vi "VPI_Thresholds.vi"(0 "Circle Mask":bool, 2 "mask":sgl[][](array[numeric]), 4 "GThresholds":T1={"Vel Range"={1.4018691588785046, 50.0}, "PFlow Range"={22.429906542056074, 90.28037383177569}, "IQ Range"={28.037383177570092, 102.05607476635514}, "ShortLag"={33.08411214953271, 88.59813084112149}, "Mean Pow"={0.0, 41.12149532710281}, "powT"={0.0, 41.12149532710281}, "varT"={0.0, 41.12149532710281}} {"varT" scale=0.0..100.0; "powT" scale=0.0..100.0; "Mean Pow" scale=0.0..100.0; "ShortLag" scale=0.0..120.0; "IQ Range" scale=-25.0..120.0; "PFlow Range" scale=0.0..120.0; "Vel Range" scale=-1.0..150.0}, 6 "Datea items":T8={"Vector Refnum"=refnum, "Vector Image"=refnum, "Data Path"=path "", "abs(IQ)"=[], "Vector Complex"=[], "pow"=[], "Dimensions"={"xdim"=0.0, "ydim"=0.0, "zdim"=0.0, "skip"=0.0, "ensembleC"=0.0, "ensembleVar\n"=0.0, "#tx"=0.0, "#Rx"=0.0, "deltaX"=0.0, "deltaY"=0.0, "x start"=0.0, "ystart"=0.0}, "vars short lag"=[], "mean pow "=[], "mean var"=[], "Color Dop Refnum"=refnum, "Color Dop Image"=refnum, "Number of vector"=0, "Number of Doppler Frames"=0, "Vector Mag"=[], "abs(IQ) SVD"=[], "powT"=[], "varT"=[], "output cluster 2"={"header info"={"Header"="", "Head length"=0}, "A/D info"={"# rf points per line"=0, "# lines per scan"=0, "sample rate MHz"=0, "# A/D bits"=0, "# bytes per A/D"=0, "TGC Flag"=0, "A/D Type"=""}, "Tranducer Info"={"bandwidth"=0.0, "center freq"=0.0, "start freq"=0.0, "ID"=0}, "Scan Info"={"delay"=0.0, "pivot distance"=0.0, "sector scan angle"=0.0, "operator"="", "Scan Mode"="", "location"=""}, "Time/Date Info"={"date"="", "time"=""}, "RF Info"={"RF file name"="", "RF file att"="", "RF cal file name"="", "RF cal file att"=""}, "Patient Info"={"ID"="", "extended ID"="", "age"=0, "sex"="", "previously\nscanned"="", "PSA"=0.0, "LOS"=1, "Ethnicty 2"=3, "Race"=3}, "Tissue Type"={"organ"=0, "disease type"=0, "disease location"=0, "IQ_pts"=0, "RcvBuffer"=0, "RcvFrame"=0, "IQBuff"=0, "IQFrame"=0, "IQPage"=0}, "Votage scaling"={"Digitizer (dB)"=0.0, "Gain (dB)"=0.0, "Atten (dB)"=0.0}, "Comment"="", "Misc Info"={"avg num"=0, "c speed"=0, "Div By or SF zones"=0, "XMIT CHS"=0, "RCV CHS"=0, "Xmit angle"=0.0}, "Therapy Parameters"={"Theraputic Freq (MHz)"=0.0, "Time on (s)"=0.0, "Therapy amplitude (mV)"=0.0, "Lines Before"=0, "Lines After"=0}, "Scan Settings"={"Energy (uJ or V)"=0, "Damp (Ohm) or Fc"=0, "HP Filt (KHz)"=0, "LP Filt (MHz)"=0, "Gain (db)"=0, "prf (kHz)"=0.0, "Distance between\nscan lines (um)"=0, "Distance between\nscan planes (um)"=0, "Scan line gap (um)"=0.0, "Scan plane gap (um)"=0.0}, "Compression Parameters"={"F1 (MHz)"=0.0, "F2 (MHz)"=0.0, "% taper"=0.0, "duration"=0.0}, "Patient Info Xtra"={"First Name"="", "Last Name"="", "Notes"=""}, "ROI Box"=[0, 0, 0, 0]}, "CleanFileName"="", "velT"=[]} {"output cluster 2"."Compression Parameters"."% taper" min=50 max=1000 format="%.2f"; "output cluster 2"."Compression Parameters"."F2 (MHz)" format="%.3f"; "output cluster 2"."Compression Parameters"."F1 (MHz)" format="%.3f"; "output cluster 2"."Scan Settings"."prf (kHz)" format="%.2f"; "output cluster 2"."Therapy Parameters"."Therapy amplitude (mV)" min=50 max=1000 format="%.2f"; "output cluster 2"."Therapy Parameters"."Time on (s)" format="%.3f"; "output cluster 2"."Therapy Parameters"."Theraputic Freq (MHz)" format="%.3f"; "output cluster 2"."Patient Info"."Race" items=["Am Ind or Alaska", "Asian", "Hawaiian, Pac Isl", "Black or Afr Amer", "White", "more than one race", "unknown"]; "output cluster 2"."Patient Info"."Ethnicty 2" items=["Hispanic", "Non-Hispanic", "unknown"]; "output cluster 2"."Patient Info"."LOS" items=["1", "2", "3", "4", "5"]; "output cluster 2"."Patient Info"."PSA" format="%.1f"; "output cluster 2"."Scan Info"."delay" format="%.2f"; "output cluster 2"."Scan Info"."pivot distance" format="%.2f"; "output cluster 2"."Scan Info"."sector scan angle" format="%.2f"; "output cluster 2"."Tranducer Info"."bandwidth" format="%.2f"; "output cluster 2"."Tranducer Info"."center freq" format="%.2f"; "output cluster 2"."Tranducer Info"."start freq" format="%.2f"}, 8 "Plane":i32 min=0 step=1, 10 "No Mask?":bool, 11 "v average in":i32=1) -> (14 "Max MeanVarS":dbl, 15 "Raw data":sgl[][](graph), 16 "Outputs":T2, 18 "output cluster":T3)   [LabVIEW 2022 SP3]
uses:
  <vilib>/vision/Avi.llb/IMAQ AVI2 Refnum.ctl
  <vilib>/vision/Image Controls.llb/IMAQ Image.ctl
  VPIParams.ctl
  ViewData/-ReadEye/Header.ctl
panel:
  out "Plane Average":csg[][](array[numeric])
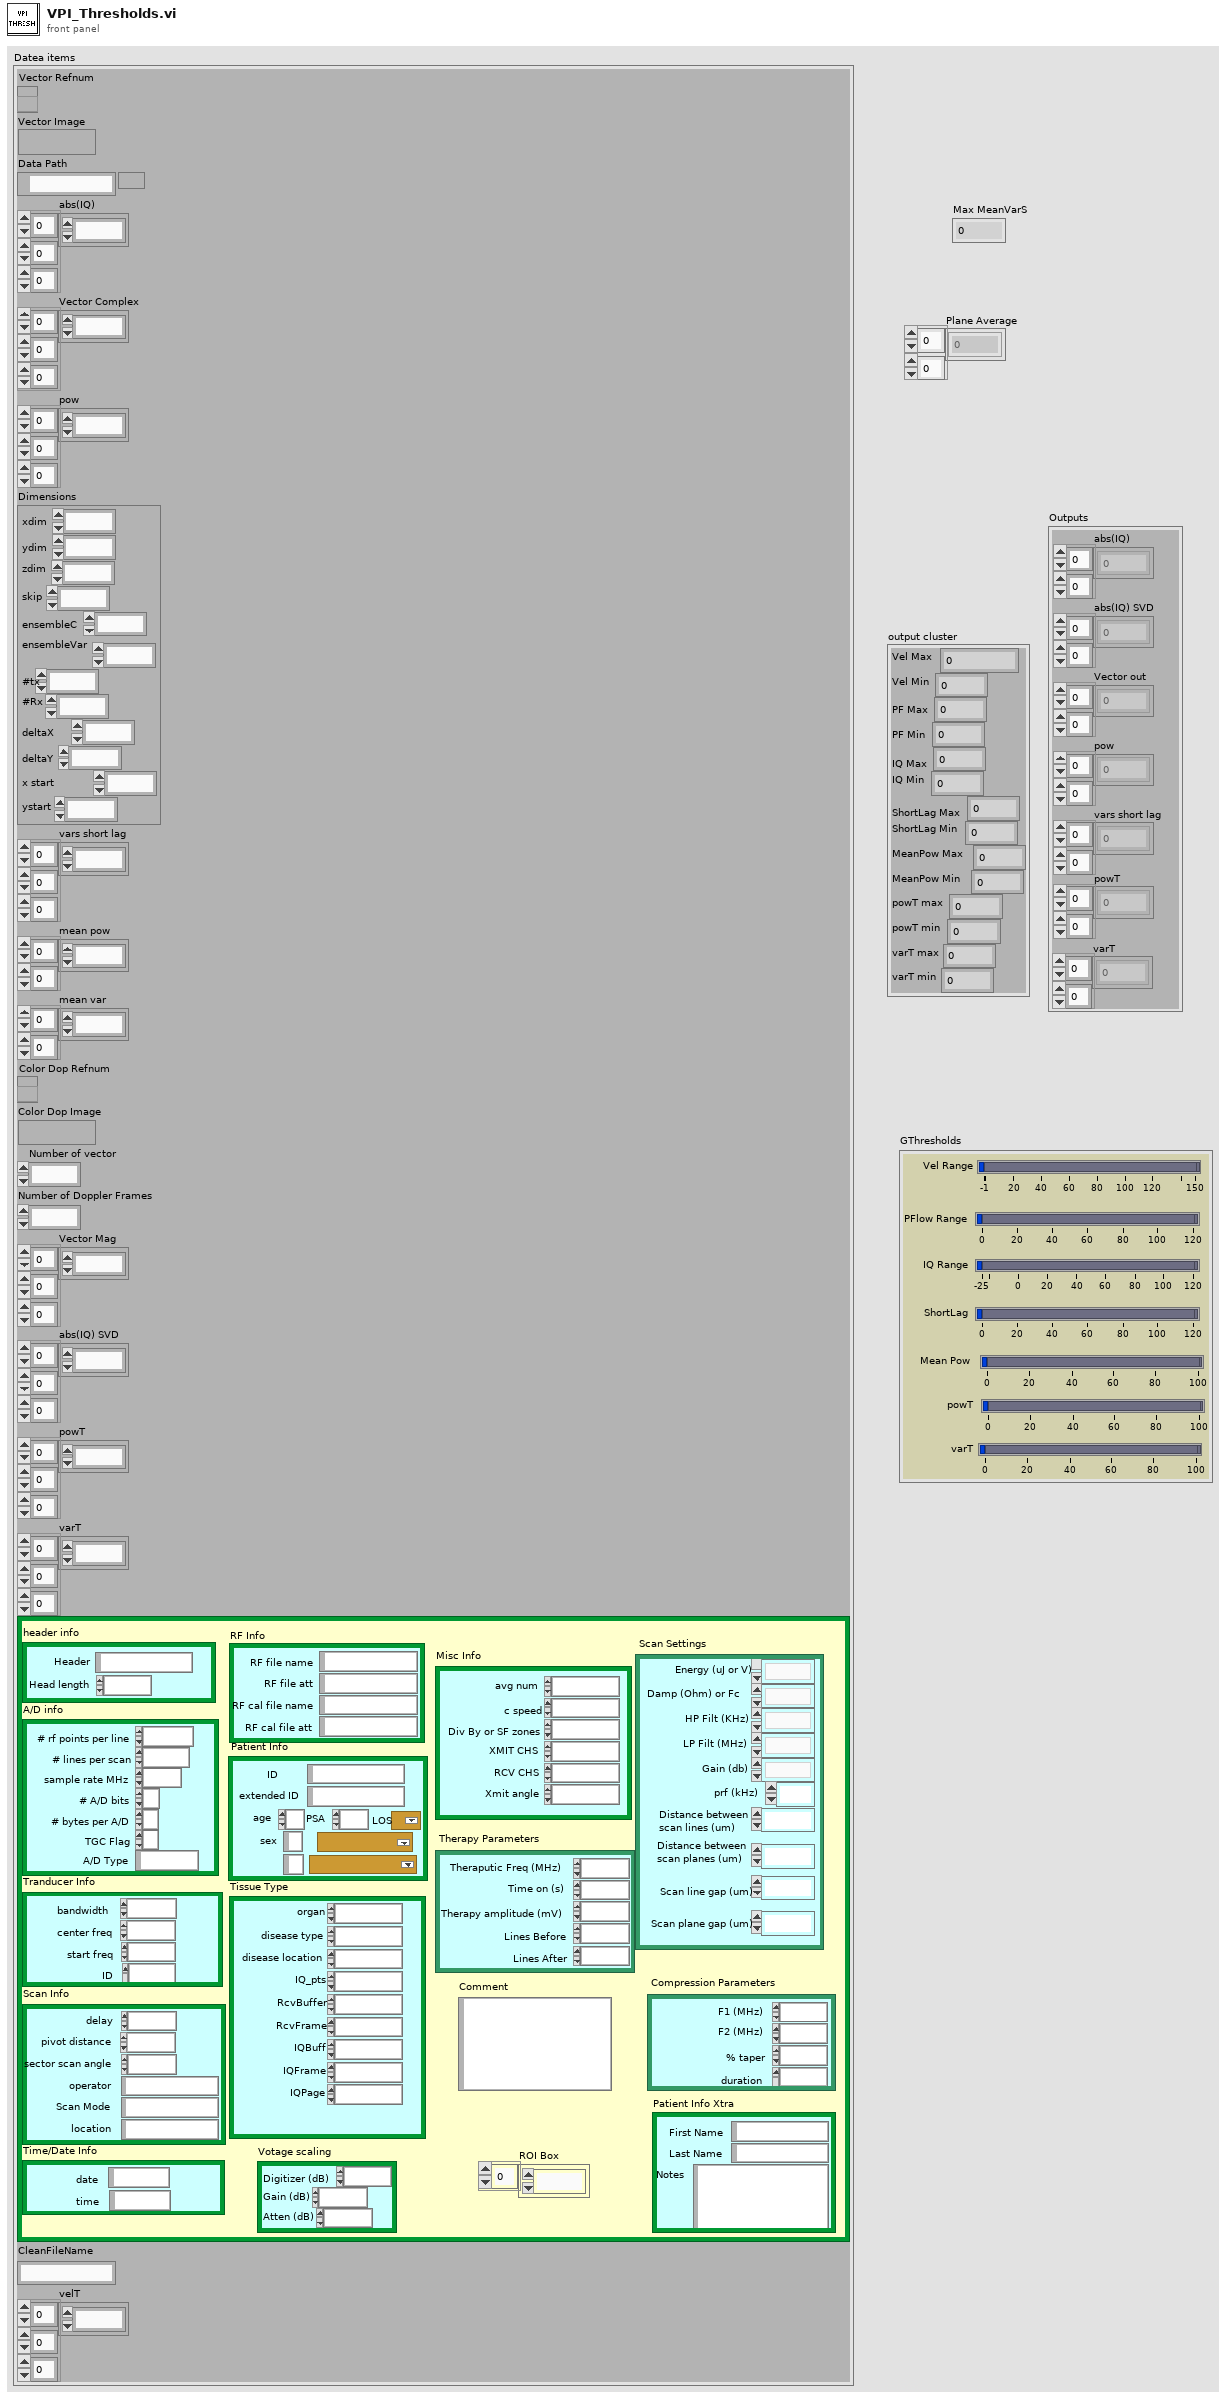
[diagram p1: front panel]
types:
  T1 = cluster{"Vel Range":cluster{dbl, dbl}, "PFlow Range":cluster{dbl, dbl}, "IQ Range":cluster{dbl, dbl}, "ShortLag":cluster{dbl, dbl}, "Mean Pow":cluster{dbl, dbl}, "powT":cluster{dbl, dbl}, "varT":cluster{dbl, dbl}}
  T2 = cluster{"abs(IQ)":sgl[][], "abs(IQ) SVD":sgl[][], "Vector out":csg[][], "pow":sgl[][], "vars short lag":sgl[][], "powT":sgl[][], "varT":sgl[][]}
  T3 = cluster{"Vel Max":sgl, "Vel Min":sgl, "PF Max":sgl, "PF Min":sgl, "IQ Max":sgl, "IQ Min":sgl, "ShortLag Max":sgl, "ShortLag Min":sgl, "MeanPow Max":sgl, "MeanPow Min":sgl, "powT max":sgl, "powT min":sgl, "varT max":sgl, "varT min":sgl}
  T4 = typedef "IMAQ AVI2 Refnum.ctl" = refnum<k20>
  T5 = typedef "IMAQ Image.ctl" = refnum<image>
  T6 = typedef "VPIParams.ctl" = cluster{"xdim":dbl, "ydim":dbl, "zdim":dbl, "skip":dbl, "ensembleC":dbl, "ensembleVar\n":dbl, "#tx":dbl, "#Rx":dbl, "deltaX":dbl, "deltaY":dbl, "x start":dbl, "ystart":dbl}
  T7 = typedef "Header.ctl" = cluster{"header info":cluster{"Header":string, "Head length":i16}, "A/D info":cluster{"# rf points per line":u16, "# lines per scan":u16, "sample rate MHz":u16, "# A/D bits":i16, "# bytes per A/D":u16, "TGC Flag":u16, "A/D Type":string}, "Tranducer Info":cluster{"bandwidth":sgl, "center freq":sgl, "start freq":sgl, "ID":i32}, "Scan Info":cluster{"delay":sgl, "pivot distance":sgl, "sector scan angle":sgl, "operator":string, "Scan Mode":string, "location":string}, "Time/Date Info":cluster{"date":string, "time":string}, "RF Info":cluster{"RF file name":string, "RF file att":string, "RF cal file name":string, "RF cal file att":string}, "Patient Info":cluster{"ID":string, "extended ID":string, "age":u16, "sex":string, "previously\nscanned":string, "PSA":sgl, "LOS":u8, "Ethnicty 2":u8, "Race":u8}, "Tissue Type":cluster{"organ":i16, "disease type":i16, "disease location":i16, "IQ_pts":u16, "RcvBuffer":u8, "RcvFrame":u16, "IQBuff":u8, "IQFrame":u16, "IQPage":u8}, "Votage scaling":cluster{"Digitizer (dB)":sgl, "Gain (dB)":sgl, "Atten (dB)":sgl}, "Comment":string, "Misc Info":cluster{"avg num":u16, "c speed":i16, "Div By or SF zones":i16, "XMIT CHS":u8, "RCV CHS":u8, "Xmit angle":sgl}, "Therapy Parameters":cluster{"Theraputic Freq (MHz)":sgl, "Time on (s)":sgl, "Therapy amplitude (mV)":sgl, "Lines Before":u16, "Lines After":u16}, "Scan Settings":cluster{"Energy (uJ or V)":u8, "Damp (Ohm) or Fc":u8, "HP Filt (KHz)":u8, "LP Filt (MHz)":u8, "Gain (db)":u8, "prf (kHz)":sgl, "Distance between\nscan lines (um)":u16, "Distance between\nscan planes (um)":u16, "Scan line gap (um)":sgl, "Scan plane gap (um)":sgl}, "Compression Parameters":cluster{"F1 (MHz)":sgl, "F2 (MHz)":sgl, "% taper":sgl, "duration":sgl}, "Patient Info Xtra":cluster{"First Name":string, "Last Name":string, "Notes":string}, "ROI Box":u16[]}
  T8 = cluster{"Vector Refnum":T4, "Vector Image":T5, "Data Path":path, "abs(IQ)":sgl[][][], "Vector Complex":csg[][][], "pow":sgl[][][], "Dimensions":T6, "vars short lag":sgl[][][], "mean pow ":sgl[][], "mean var":sgl[][], "Color Dop Refnum":T4, "Color Dop Image":T5, "Number of vector":u32, "Number of Doppler Frames":u32, "Vector Mag":sgl[][][], "abs(IQ) SVD":sgl[][][], "powT":sgl[][][], "varT":sgl[][][], "output cluster 2":T7, "CleanFileName":string, "velT":sgl[][][]}
  T9 = cluster{sgl, sgl, sgl, sgl, sgl, sgl, sgl, sgl, sgl, sgl, sgl, sgl, sgl, sgl}
  T10 = cluster{"abs(IQ)":sgl[][], "abs(IQ) SVD":sgl[][], csg[][], "pow":sgl[][], "vars short lag":sgl[][], "powT":sgl[][], "varT":sgl[][]}
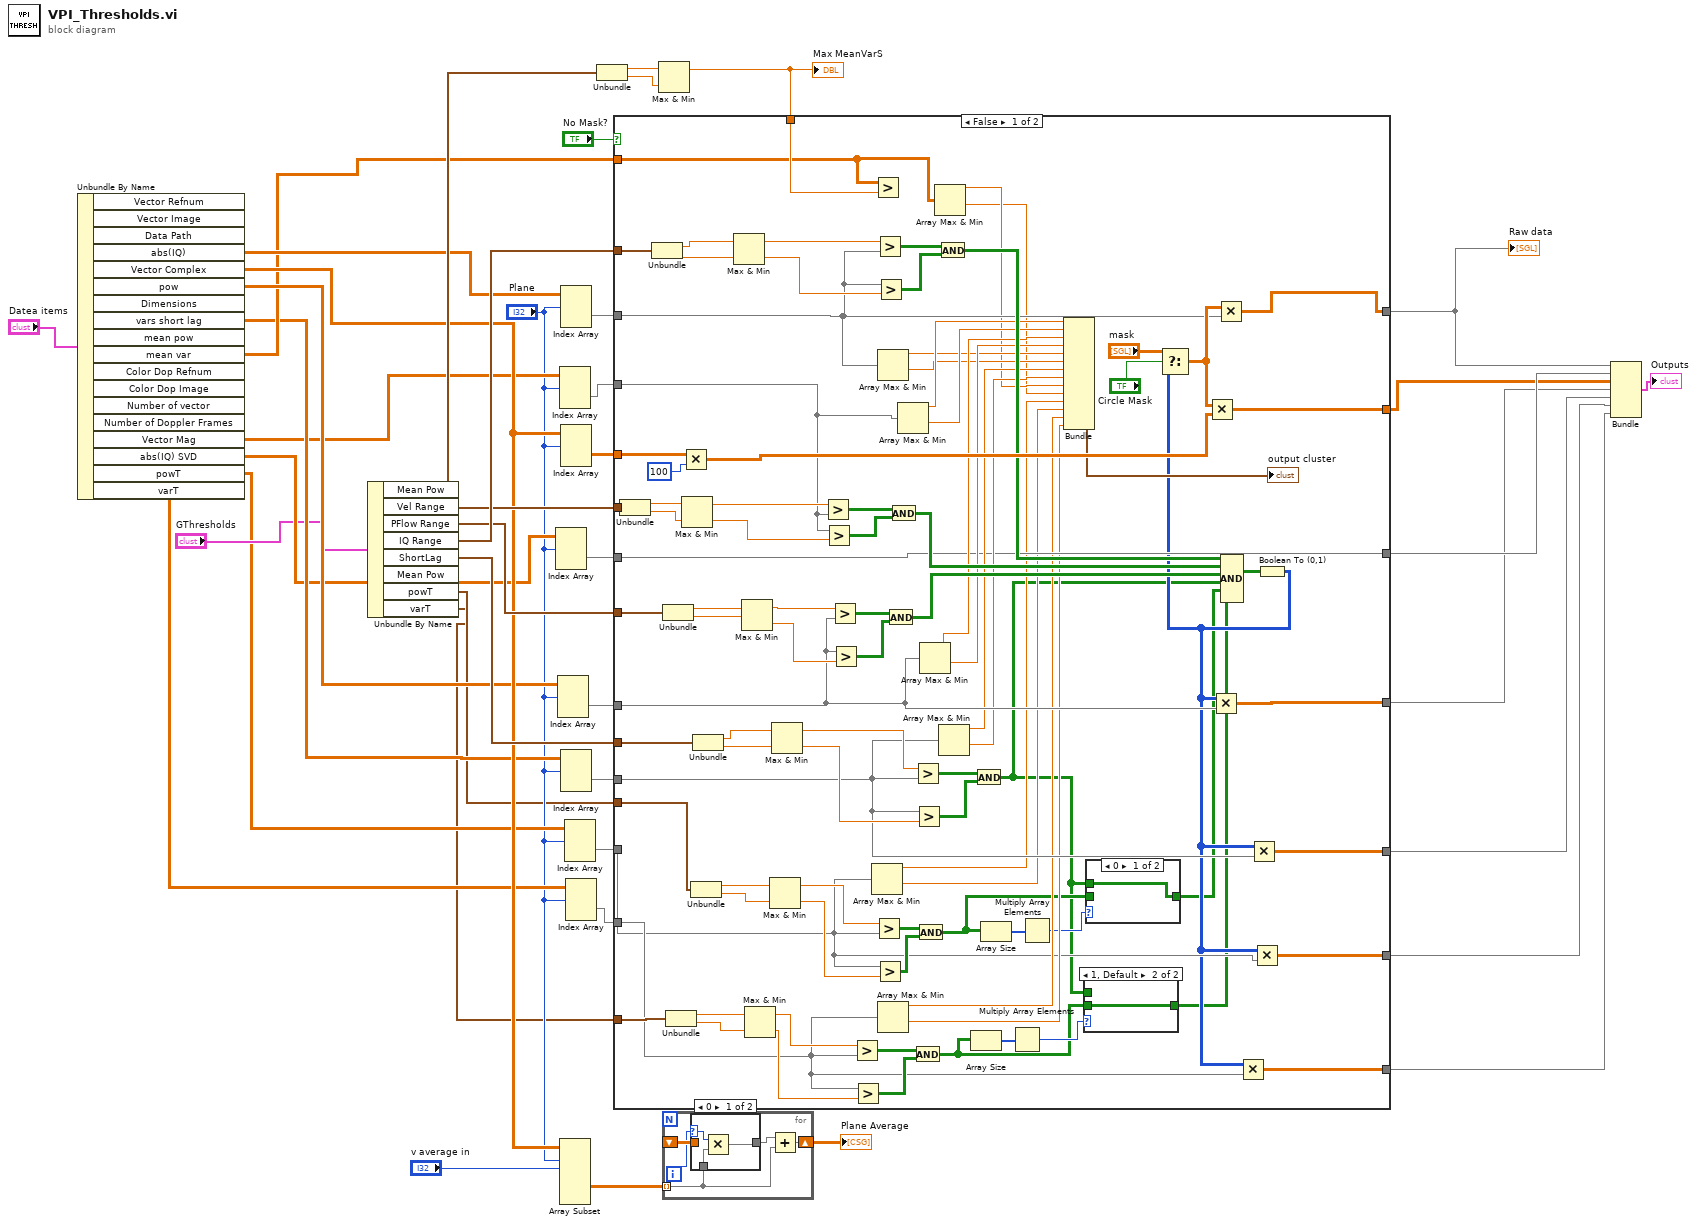
[diagram p0: block diagram]
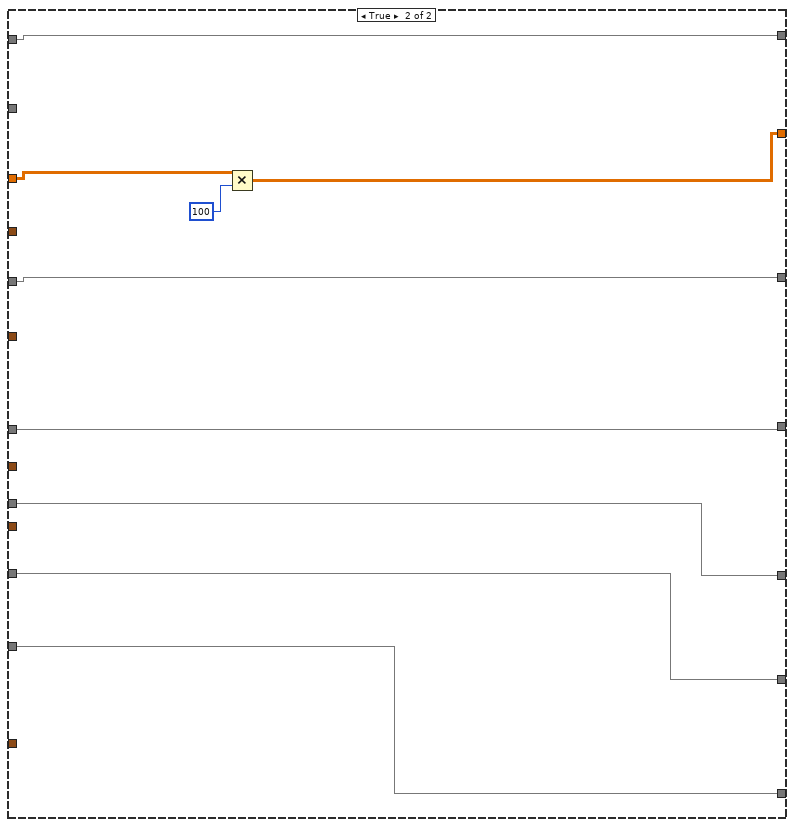
[diagram p4: hidden frame]
diagram:
  n1 = Unbundle By Name("Datea items") -> ("abs(IQ)"=w25:sgl[][][], "Vector Complex"=w24:csg[][][], "pow"=w23:sgl[][][], "vars short lag"=w21:sgl[][][], "mean var"=w22:sgl[][], "Vector Mag"=w19:sgl[][][], "abs(IQ) SVD"=w18:sgl[][][], "powT"=w10:sgl[][][], "varT"=w9:sgl[][][])  [unwired: 9 out]
  n2 = Unbundle By Name("GThresholds") -> ("Mean Pow"=w29:cluster{dbl, dbl}, "Vel Range"=w36:cluster{dbl, dbl}, "PFlow Range"=w27:cluster{dbl, dbl}, "IQ Range"=w37:cluster{dbl, dbl}, "ShortLag"=w35:cluster{dbl, dbl}, "powT"=w7:cluster{dbl, dbl}, "varT"=w6:cluster{dbl, dbl})  [unwired: 1 out]
  n3 = Index Array(array=w18, index (dim 0)="Plane") -> (element=w17:sgl[][])  [unwired: 2 in]
  n4 = Index Array(array=w23, index (dim 0)="Plane") -> (element=w33:sgl[][])  [unwired: 2 in]
  n5 = Index Array(array=w19, index (dim 0)="Plane") -> (element=w20:sgl[][])  [unwired: 2 in]
  n6 = Array Subset(array=w24, index (dim 0)="Plane", length (dim 0)="v average in") -> (w41:csg[][][])  [unwired: 4 in]
  n7 = Index Array(array=w25, index (dim 0)="Plane") -> (element=w38:sgl[][])  [unwired: 2 in]
  n8 = Index Array(array=w24, index (dim 0)="Plane") -> (element=w39:csg[][])  [unwired: 2 in]
  n9 = Index Array(array=w21, index (dim 0)="Plane") -> (element=w34:sgl[][])  [unwired: 2 in]
  n10 = Index Array(array=w10, index (dim 0)="Plane") -> (element=w5:sgl[][])  [unwired: 2 in]
  n11 = Index Array(array=w9, index (dim 0)="Plane") -> (element=w4:sgl[][])  [unwired: 2 in]
  n12 = Unbundle(w29) -> (w31:dbl, w32:dbl)
  n13 = Max & Min(x=w31, y=w32) -> (max(x,y)=w30:dbl)  [unwired: 1 out]
  "Max MeanVarS" <- w30
  n14 = case shown="False" "No Mask?" {
    tunnel: [w75 w147] -> w16
    tunnel: w39 -> [w117 w144]
    tunnel: [w115 w143] -> w12
    tunnel: w38 -> [w92 w147]
    tunnel: w37 -> [w106 _]
    tunnel: w36 -> [w105 _]
    tunnel: w27 -> [w104 _]
    tunnel: w35 -> [w97 _]
    tunnel: [w96 w146] -> w13
    tunnel: w34 -> [w91 w146]
    tunnel: w33 -> [w89 w145]
    tunnel: [w95 w145] -> w14
    tunnel: w30 -> [w94 _]
    tunnel: w20 -> [w90 _]
    tunnel: w22 -> [w88 _]
    tunnel: [w76 w141] -> w15
    tunnel: w17 -> [w76 w141]
    tunnel: w7 -> [w68 _]
    tunnel: w6 -> [w61 _]
    tunnel: w5 -> [w53 w140]
    tunnel: w4 -> [w58 w139]
    tunnel: [w60 w140] -> w3
    tunnel: [w59 w139] -> w2
    frame False {
      n15 = Unbundle(w105) -> (w132:dbl, w131:dbl)
      n16 = Unbundle(w106) -> (w109:dbl, w108:dbl)
      n17 = Unbundle(w104) -> (w134:dbl, w133:dbl)
      n18 = Unbundle(w61) -> (w67:dbl, w66:dbl)
      n19 = Multiply(x=w117, y=100) -> (x*y=w116:csg[][])
      n20 = Max & Min(x=w132, y=w131) -> (max(x,y)=w124:dbl, min(x,y)=w123:dbl)
      n21 = Unbundle(w68) -> (w74:dbl, w73:dbl)
      n22 = Unbundle(w97) -> (w103:dbl, w102:dbl)
      n23 = Max & Min(x=w109, y=w108) -> (max(x,y)=w111:dbl, min(x,y)=w110:dbl)
      n24 = Max & Min(x=w134, y=w133) -> (max(x,y)=w130:dbl, min(x,y)=w129:dbl)
      n25 = Max & Min(x=w67, y=w66) -> (max(x,y)=w65:dbl, min(x,y)=w64:dbl)
      n26 = Max & Min(x=w74, y=w73) -> (max(x,y)=w72:dbl, min(x,y)=w71:dbl)
      n27 = Max & Min(x=w103, y=w102) -> (max(x,y)=w101:dbl, min(x,y)=w100:dbl)
      n28 = Greater?(x=w124, y=w90) -> (0:w125:bool[][])
      n29 = Greater?(x=w90, y=w123) -> (0:w126:bool[][])
      n30 = Greater?(x=w130, y=w89) -> (0:w127:bool[][])
      n31 = Greater?(x=w89, y=w129) -> (0:w128:bool[][])
      n32 = Greater?(x=w65, y=w58) -> (0:w62:bool[][])
      n33 = Greater?(x=w58, y=w64) -> (0:w63:bool[][])
      n34 = Array Max & Min(array=w53) -> (max value=w57:sgl, min value=w56:sgl)  [unwired: 2 out]
      n35 = Greater?(x=w88, y=w94) -> ()  [unwired: 1 out]
      n36 = Greater?(x=w72, y=w53) -> (0:w69:bool[][])
      n37 = Greater?(x=w111, y=w92) -> (0:w112:bool[][])
      n38 = Greater?(x=w53, y=w71) -> (0:w70:bool[][])
      n39 = Greater?(x=w92, y=w110) -> (0:w113:bool[][])
      n40 = Array Max & Min(array=w92) -> (max value=w83:sgl, min value=w82:sgl)  [unwired: 2 out]
      n41 = Array Max & Min(array=w58) -> (max value=w55:sgl, min value=w54:sgl)  [unwired: 2 out]
      n42 = And(x=w127, y=w128) -> (x .and. y?=w121:bool[][])
      n43 = And(x=w125, y=w126) -> (x .and. y?=w122:bool[][])
      n44 = Array Max & Min(array=w90) -> (max value=w87:sgl, min value=w86:sgl)  [unwired: 2 out]
      n45 = Greater?(x=w101, y=w91) -> (0:w98:bool[][])
      n46 = And(x=w62, y=w63) -> (x .and. y?=w45:bool[][])
      n47 = Greater?(x=w91, y=w100) -> (0:w99:bool[][])
      n48 = And(x=w69, y=w70) -> (x .and. y?=w48:bool[][])
      n49 = Array Max & Min(array=w89) -> (max value=w85:sgl, min value=w84:sgl)  [unwired: 2 out]
      n50 = Array Max & Min(array=w88) -> (max value=w79:sgl, min value=w78:sgl)  [unwired: 2 out]
      n51 = And(x=w112, y=w113) -> (x .and. y?=w107:bool[][])
      n52 = Array Max & Min(array=w91) -> (max value=w81:sgl, min value=w80:sgl)  [unwired: 2 out]
      n53 = Array Size(array=w45) -> (size(s)=w47:i32[])
      n54 = And(x=w98, y=w99) -> (x .and. y?=w44:bool[][])
      n55 = Array Size(array=w48) -> (size(s)=w52:i32[])
      n56 = Multiply Array Elements(1:w47) -> (0:w46:i32)
      n57 = Multiply Array Elements(1:w52) -> (0:w50:i32)
      n58 = Bundle(w87, w86, w85, w84, w83, w82, w81, w80, w79, w78, w57, w56, w55, w54) -> (→"output cluster":T9)  [unwired: 1 in]
      n59 = case shown="1, Default" w46 {
        tunnel: [w135 w136] -> w43
        tunnel: w45 -> [_ w136]
        tunnel: w44 -> [w135 _]
        frame 0 {
        }
        frame 1, Default {
        }
      }
      n60 = case shown="0" w50 {
        tunnel: [w137 w138] -> w49
        tunnel: w48 -> [_ w138]
        tunnel: w44 -> [w137 _]
        frame 0 {
        }
        frame 1, Default {
        }
      }
      n61 = Compound Arithmetic op=AND(w107, w122, w121, w44, w49, w43) -> (w93:bool[][])
      n62 = Boolean To (0,1)(Boolean=w93) -> (0, 1=w51:i16[][])
      n63 = Select(t="mask", s="Circle Mask", f=w51) -> (s? t:f=w119:sgl[][])
      n64 = Multiply(x=w119, y=w116) -> (x*y=w115:csg[][])
      n65 = Multiply(x=w51, y=w89) -> (x*y=w95:sgl[][])
      n66 = Multiply(x=w119, y=w92) -> (x*y=w75:sgl[][])
      n67 = Multiply(x=w51, y=w58) -> (x*y=w59:sgl[][])
      n68 = Multiply(x=w51, y=w91) -> (x*y=w96:sgl[][])
      n69 = Multiply(x=w51, y=w53) -> (x*y=w60:sgl[][])
    }
    frame True {
      n70 = Multiply(x=w144, y=100) -> (x*y=w143:csg[][])
    }
  }
  "Raw data" <- w16
  n71 = for {
    tunnel: w41 -> [w148] mode=indexing
    shift-right: [w152] -> w40
    shift-left: _ -> [w150]
    i -> [w149]
    n72 = case shown="0" w149 {
      selector: w149 -> [w155 _]
      tunnel: [w154 w156] -> w151
      tunnel: w150 -> [_ w156]
      tunnel: w148 -> [w153 _]
      frame 0 {
        n73 = Multiply(x=w155, y=w153) -> (x*y=w154:csg[][])
      }
      frame 1, Default {
      }
    }
    n74 = Add(x=w151, y=w148) -> (x+y=w152:csg[][])
  }
  "Plane Average" <- w40
  n75 = Bundle("abs(IQ)"=w16, "abs(IQ) SVD"=w15, w12, "pow"=w14, "vars short lag"=w13, "powT"=w3, "varT"=w2) -> (→"Outputs":T10)  [unwired: 1 in]
